vi "OpenNetworkStreamReader.vi"(6 "connection timeout":i32=-1, 7 "reader buffer size":i32, 8 "error in (no error)":errorcluster, 9 "writer url":string, 10 "reader name":string, 11 "NetworkStreamReader in":refnum<class "NetworkStreamReader.lvclass">) -> (0 "error out":errorcluster, 1 "Initialized?":bool, 2 "Reader Endpoint":refnum<k21>, 3 "NetworkStreamReader out":refnum<class "NetworkStreamReader.lvclass">)   [LabVIEW 2011, in "NetworkStreamReader.lvclass"]
doc: "Opens a network stream reader endpoint. This VI persistently tries to open the connection until it is successful or the e-stop is triggered."
uses:
  NetworkStreamReader.lvclass
  Shared/message.ctl
  NetworkStreamReader.lvclass/NetworkStreamReader.ctl
  2-Think/2 Globals/2 Global.vi
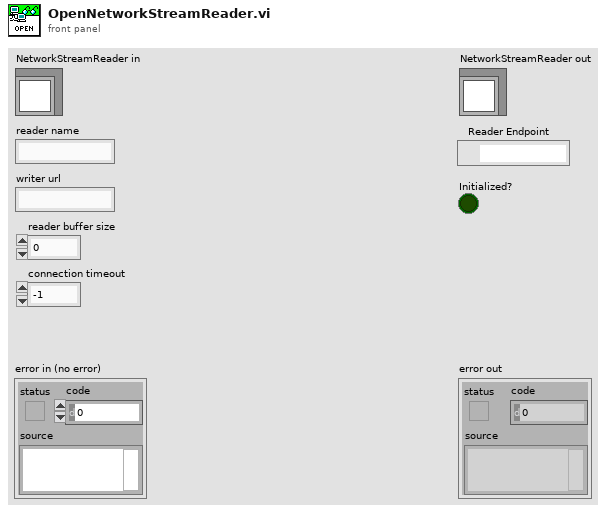
[diagram p1: front panel]
types:
  T1 = typedef "message.ctl" = cluster{"Data":variant, "Time since start (s)":dbl}
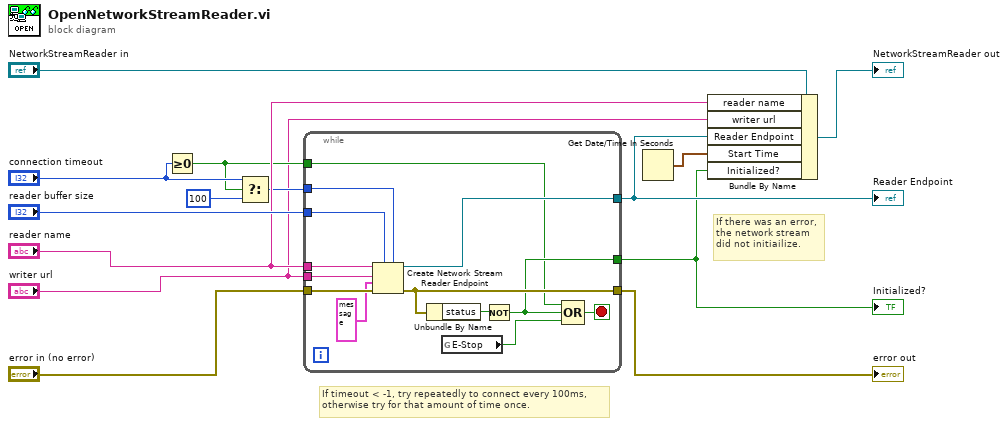
[diagram p0: block diagram]
diagram:
  # "If timeout < -1, try repeatedly to connect every 100ms,\notherwise try for that amount of time once."
  # "If there was an error,\nthe network stream\ndid not initiailize."
  n1 = Greater Or Equal To 0?(x="connection timeout") -> (x >= 0?=w4:bool)
  n2 = Select(t="connection timeout", s=w4, f=100 ("t")) -> (s? t:f=w3:i32)
  n3 = while {
    tunnel: "error in (no error)" -> [w27]
    tunnel: "reader buffer size" -> [w26]
    tunnel: [w22] -> w13
    tunnel: "reader name" -> [w25]
    tunnel: "writer url" -> [w24]
    tunnel: [w20] -> w8
    tunnel: [w18] -> w5
    tunnel: w4 -> [w16]
    tunnel: w3 -> [w15]
    stop <- w17 stop-if-true
    n4 = Create Network Stream Reader Endpoint(5:w15, 7:w26, 8:w27, 9:T1 {"Data"=variant, "Time since start (s)"=0.0} ("variant"), 10:w24, 11:w25) -> (0:w22:errorcluster, 3:w20:refnum<k21>)
    n5 = Unbundle By Name(w22) -> ("status"=w21:bool)
    n6 = global read "2 Global.vi" "E-Stop"() -> (w19:bool)
    n7 = Not(x=w21) -> (.not. x?=w18:bool)
    n8 = Compound Arithmetic op=OR(w16, w18, w19) -> (w17:bool)
  }
  "error out" <- w13
  "Reader Endpoint" <- w8
  "Initialized?" <- w5
  n9 = Get Date/Time In Seconds() -> (seconds since 1Jan1904=w6:timestamp)
  n10 = Bundle By Name(cluster="NetworkStreamReader in", "reader name"="reader name", "writer url"="writer url", "Reader Endpoint"=w8, "Start Time"=w6, "Initialized?"=w5) -> (→"NetworkStreamReader out":refnum<class "NetworkStreamReader.lvclass">)
